vi "slscswitch Relay Control.vi"(8 "error in (no error)":errorcluster, 9 "relay action (Close Relay)":T1=enum."Close Relay", 10 "relay name":string, 11 "SLSC Switch in":refnum<class "SLSC Switch.lvclass">) -> (0 "error out":errorcluster, 3 "SLSC Switch out":refnum<class "SLSC Switch.lvclass">)   [LabVIEW 2015, in "SLSC Switch.lvclass"]
uses:
  SLSC Switch.lvclass
  Relay Action.ctl
  SLSC Switch.lvclass/SLSC Switch.ctl
  <vilib>/SLSC/Set Device Property (Bool).vi
  <vilib>/SLSC/Commit Properties for Devices.vi
  <vilib>/SLSC/Execute Device Command.vi
  Route Manager/Route Manager.lvclass
  <vilib>/SLSC/SLSC.lvlib
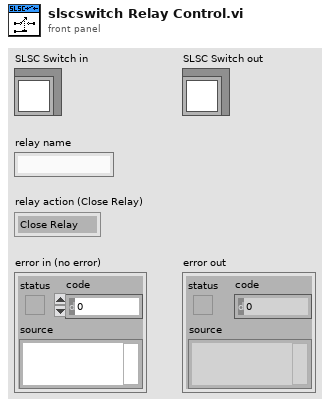
[diagram p1: front panel]
types:
  T1 = typedef "SLSC Switch.lvclass/Relay Action.ctl" = enum16{"Open Relay", "Close Relay"}
  T2 = typedef "Route Manager.lvclass/Relay Info.ctl" = cluster{"property":refnum<k21>, "command":refnum<k21>}
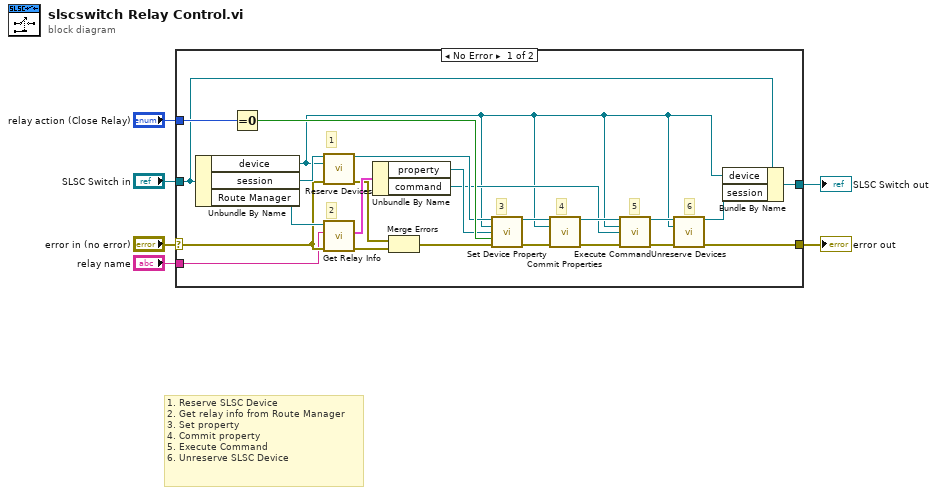
[diagram p0: block diagram]
diagram:
  # "1. Reserve SLSC Device\n2. Get relay info from Route Manager\n3. Set property\n4. Commit property\n5. Execute Command\n6. Unreserve SLSC Device"
  n1 = case shown="No Error" "error in (no error)" {
    selector: "error in (no error)" -> [w10 w32]
    tunnel: [w16 w32] -> w5
    tunnel: [w14 w31] -> w3
    tunnel: "SLSC Switch in" -> [w15 w31]
    tunnel: "relay action (Close Relay)" -> [w28 _]
    tunnel: "relay name" -> [w7 _]
    frame No Error {
      # "6"
      # "5"
      # "4"
      # "3"
      # "2"
      # "1"
      n2 = Unbundle By Name(w15) -> ("device"=w13:refnum<k21>, "session"=w29:refnum<k21>, "Route Manager"=w30:refnum<class "Route Manager.lvclass">)
      n3 = Equal To 0?(x=w28) -> (x = 0?=w27:bool)
      n4 = call <vilib>:"Reserve Devices.vi"("session in"=w29, "devices"=w13, "error in (no error)"=w10) -> ("session out"=w26:refnum<k21>, "error out"=w11:errorcluster)  [unwired: 11 in]
      n5 = call "Get Relay Info.vi"("error in (no error)"=w10, "relay string"=w7, "Route Manager in"=w30) -> ("error out"=w9:errorcluster, "relay info"=w25:T2)  [unwired: 7 in]
      n6 = Unbundle By Name(w25) -> ("property"=w24:refnum<k21>, "command"=w20:refnum<k21>)
      n7 = Merge Errors(w11, w9) -> (w8:errorcluster)
      n8 = call-poly <vilib>:"Set Device Property.vi"("session in"=w26, "devices"=w13, "property"=w24, "property value"=w27, "error in (no error)"=w8) -> ("session out"=w23:refnum<k21>, "error out"=w22:errorcluster)  [unwired: 9 in]
      n9 = call-poly <vilib>:"Commit Properties.vi"("session in"=w23, "devices"=w13, "error in (no error)"=w22) -> ("session out"=w21:refnum<k21>, "error out"=w19:errorcluster)  [unwired: 11 in]
      n10 = call-poly <vilib>:"Execute Command.vi"("session in"=w21, "devices"=w13, "command"=w20, "error in (no error)"=w19) -> ("session out"=w18:refnum<k21>, "error out"=w17:errorcluster)  [unwired: 10 in]
      n11 = call <vilib>:"Unreserve Devices.vi"("session in"=w18, "devices"=w13, "error in (no error)"=w17) -> ("session out"=w12:refnum<k21>, "error out"=w16:errorcluster)  [unwired: 11 in]
      n12 = Bundle By Name(cluster=w15, "device"=w13, "session"=w12) -> (w14:refnum<class "SLSC Switch.lvclass">)
    }
    frame Error {
    }
  }
  "error out" <- w5
  "SLSC Switch out" <- w3
